vi "formatIntoTable.vi"(8 "error in (no error)":errorcluster, 11 "TransactionList in":refnum<class "TransactionList.lvclass">) -> (0 "error out":errorcluster, 2 "Table Row":string[][](array[string]), 3 "TransactionList out":refnum<class "TransactionList.lvclass">)   [LabVIEW 2018, in "TransactionList.lvclass"]
uses:
  TransactionList.lvclass
  TransactionList.lvclass/TransactionList.ctl
  Transaction/Transaction.lvclass
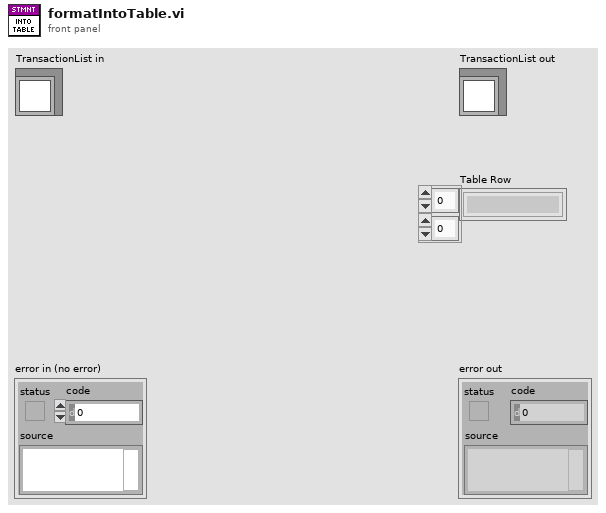
[diagram p1: front panel]
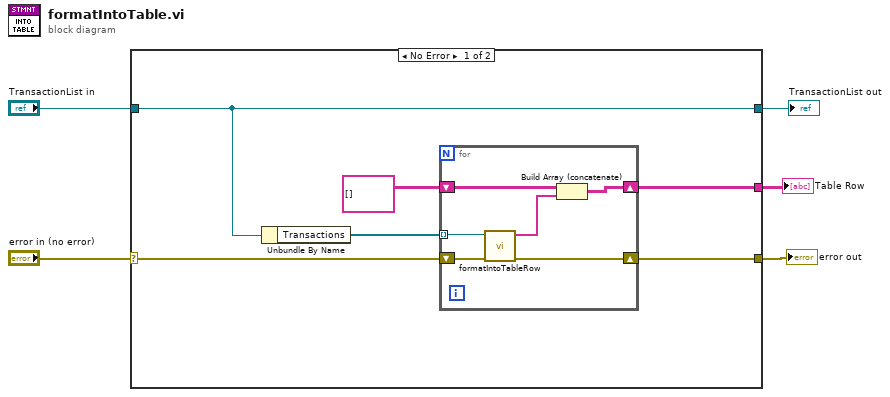
[diagram p0: block diagram]
diagram:
  n1 = case shown="No Error" "error in (no error)" {
    selector: "error in (no error)" -> [w8 w19]
    tunnel: [w11 w19] -> w4
    tunnel: [w10 w18] -> w2
    tunnel: "TransactionList in" -> [w10 w18]
    tunnel: [w6 _] -> w1
    frame No Error {
      n2 = Unbundle By Name(w10) -> ("Transactions"=w9:refnum<class "Transaction.lvclass">[])
      n3 = for {
        tunnel: w9 -> [w17] mode=indexing
        shift-right: [w15] -> w11
        shift-left: w8 -> [w16]
        shift-right: [w12] -> w6
        shift-left: string[][] [] ("Table Row") -> [w14]
        n4 = call "formatIntoTableRow.vi"("error in (no error)"=w16, "Transaction in"=w17) -> ("error out"=w15:errorcluster, "Table Row"=w13:string[])  [unwired: 8 in]
        n5 = Build Array (concatenate)(w14, w13) -> (w12:string[][])
      }
    }
    frame Error {
    }
  }
  "error out" <- w4
  "TransactionList out" <- w2
  "Table Row" <- w1
